vi "potFieldEnemyRadiusByVel.vi"(4 "min multiplier(enemy)":dbl(slide)=2.9591836734693877 scale=0.0..10.0, 6 "max multiplier(enemy)":dbl(slide)=2.9591836734693877 scale=0.0..10.0, 8 "error in (no error)":errorcluster, 9 "min influence radius(enemy)":dbl=1000.0 format="%#_13g", 10 "max influence radius(enemy)":dbl=1000.0 format="%#_13g", 11 "Robot in":refnum<class "Robot.lvclass">) -> (0 "error out":errorcluster, 1 "enemy multiplier":dbl, 2 "enemy influence radius":dbl, 3 "Robot out":refnum<class "Robot.lvclass">)   [LabVIEW 2020, in "Robot.lvclass"]
uses:
  Robot.lvclass
  <vilib>/Analysis/_algsub.llb/Real Vector Norm.vi
  <vilib>/Analysis/NI_AALPro.lvlib
  Utilities_class/Utilities.lvclass
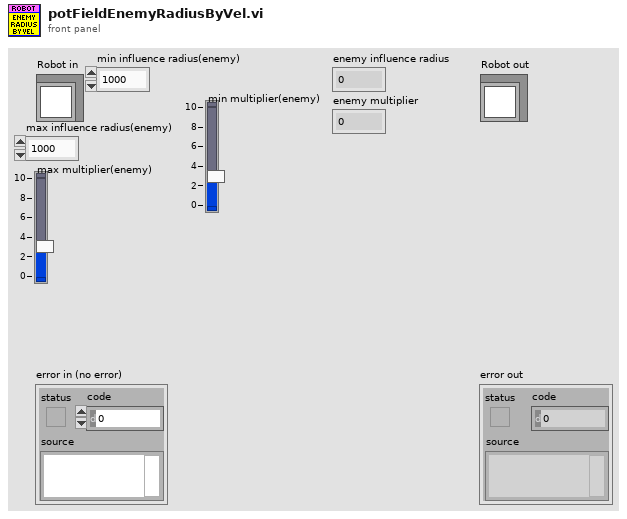
[diagram p1: front panel]
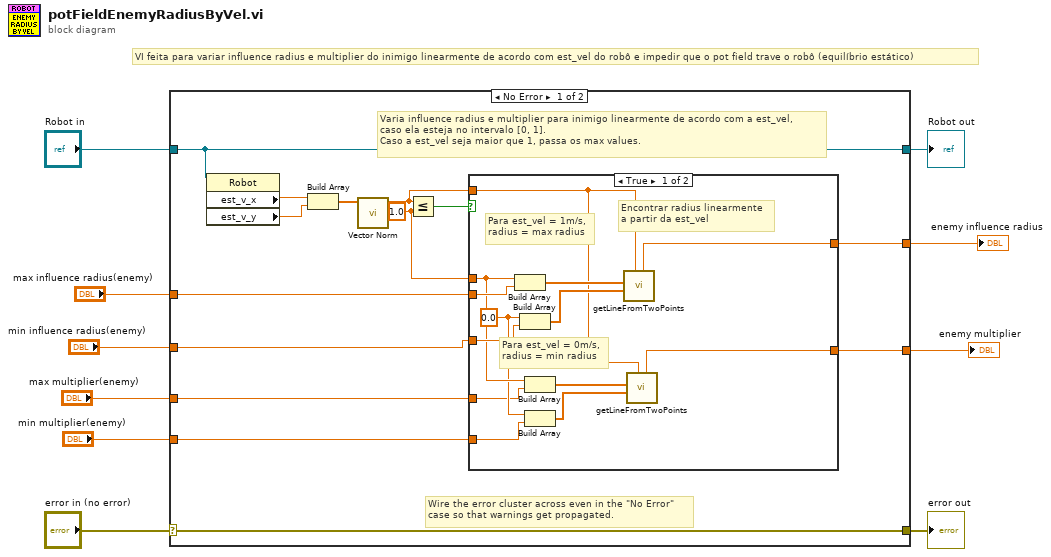
[diagram p0: block diagram]
diagram:
  # "VI feita para variar influence radius e multiplier do inimigo linearmente de acordo com est_vel do robô e impedir que o pot field trave o robô (equilíbrio estático)"
  n1 = case shown="No Error" "error in (no error)" {
    selector: "error in (no error)" -> [w24 w41]
    tunnel: [w24 w41] -> w9
    tunnel: [w23 w40] -> w7
    tunnel: "Robot in" -> [w23 w40]
    tunnel: "max influence radius(enemy)" -> [w17 _]
    tunnel: "min influence radius(enemy)" -> [w16 _]
    tunnel: [w14 _] -> w4
    tunnel: "max multiplier(enemy)" -> [w13 _]
    tunnel: "min multiplier(enemy)" -> [w12 _]
    tunnel: [w11 _] -> w1
    frame No Error {
      w18 = 1.0 ("y")
      # "Varia influence radius e multiplier para inimigo linearmente de acordo com a est_vel,\ncaso ela esteja no intervalo [0, 1].\nCaso a est_vel seja maior que 1, passa os max values."
      # "Wire the error cluster across even in the \"No Error\"\ncase so that warnings get propagated."
      n2 = property class="Robot"(reference=w23) -> ("est_v_x"=w22:dbl, "est_v_y"=w21:dbl)  [unwired: 1 in, 2 out]
      n3 = Build Array(w22, w21) -> (w20:dbl[])
      n4 = call-poly <vilib>:"Vector Norm.vi"("Input Vector"=w20) -> ("norm"=w15:dbl)  [unwired: 9 in, 1 out]
      n5 = Less Or Equal?(x=w15, y=w18) -> (x <= y?=w19:bool)
      n6 = case shown="True" w19 {
        tunnel: w18 -> [w32 _]
        tunnel: w17 -> [w37 w39]
        tunnel: w16 -> [w36 _]
        tunnel: w15 -> [w26 _]
        tunnel: [w33 w39] -> w14
        tunnel: w13 -> [w30 w38]
        tunnel: w12 -> [w29 _]
        tunnel: [w25 w38] -> w11
        frame True {
          w31 = 0.0 ("element")
          # "Encontrar radius linearmente\na partir da est_vel"
          # "Para est_vel = 0m/s,\nradius = min radius"
          # "Para est_vel = 1m/s,\nradius = max radius"
          n7 = Build Array(w32, w37) -> (w35:dbl[])
          n8 = Build Array(w31, w36) -> (w34:dbl[])
          n9 = Build Array(w32, w30) -> (w28:dbl[])
          n10 = Build Array(w31, w29) -> (w27:dbl[])
          n11 = call "getLineFromTwoPoints.vi"("x informed (optional)"=w26, "Point 2"=w34, "Point 1"=w35) -> ("y to x informed (opitional)"=w33:dbl)  [unwired: 4 in, 4 out]
          n12 = call "getLineFromTwoPoints.vi"("x informed (optional)"=w26, "Point 2"=w27, "Point 1"=w28) -> ("y to x informed (opitional)"=w25:dbl)  [unwired: 4 in, 4 out]
        }
        frame False {
        }
      }
    }
    frame Error {
    }
  }
  "error out" <- w9
  "Robot out" <- w7
  "enemy influence radius" <- w4
  "enemy multiplier" <- w1
